vi "Stuckbead Scan and Auto Save_YCC.vi"(8 "File name add to the end":string="h0", 9 "Scan Range  (um)":dbl=2.0 format="%.3f", 10 "Save Data?":bool, 11 "Axis (XYZ)":enum16{"x", "y", "z"}(ring)) -> ()   [LabVIEW 2014]
uses:
  Main-Stage-PI/(Global) Current handle and LaserPower_YCC.vi
  <vilib>/Analysis/polynomials.llb/Scalar Polynomial Evaluation (DBL).vi
  <vilib>/Analysis/NI_AALPro.lvlib
panel:
  in  "Filter type":T1(ring)=enum."Moving-window avg"
  out "delta xBead (nm)":dbl[](array[numeric])
  out "Bead Position (nm)":dbl[](array[numeric])
  in  "Stuckbead path (dialog if empty)":path=path "D:/Calibration-Stuckbead-Scan/20181030/2/034619-x-Stuckbead Scan-20.00-step 5.00 nm-QPD height 0.814-h0.txt"
  in  "Who's Data":T2(ring)
  out "step size (nm)":dbl
  out "QPD height for tether (V)":dbl
  in  "Enum":enum16{"parity method", "max-min method"}(ring)=enum."max-min method"
  out "mean QPD":dbl
  out "Positon Start scan point (um)":dbl
  out "Filtered QPD data":dbl[](array[numeric])
  out "Filtered Stage Array":dbl[](array[numeric])
  out "Running time":dbl
  in  "Move to new Center?":bool=TRUE
  in  "no record \nscan rate  (um/s)":dbl=4.0
  out "need time":dbl
  out "True rate?":bool
  out "Sample points want to record":dbl
  out "Center (um)":dbl
  out "Move to":dbl
  in  "Tab Control":T3(tab)
  out "Filtered stage-QPD Graph (XY)":T4(graph)
  out "Raw+Filter stage-QPD Graph":cluster{"Raw Stage Array":dbl[], "data":dbl[]}[](graph)
  out "stage-QPD Graph":cluster{"Raw Stage Array":dbl[], "data":dbl[]}[](graph)
  in  "Avg points":i32=620
  out "Stage Array from one end to the other end":dbl[](array[numeric])
  out "total time to travel (s)":dbl
  out "Axis to Read":i32
  in  "T=+ first\nF=- first":bool
  out "Real initial position (um)":dbl format="%0.5f"
  in  "Sampling rate (Hz)":dbl=32000.0 format="%0.2f"
  in  "scan rate  (um/s)":dbl=1.0 format="%.3f"
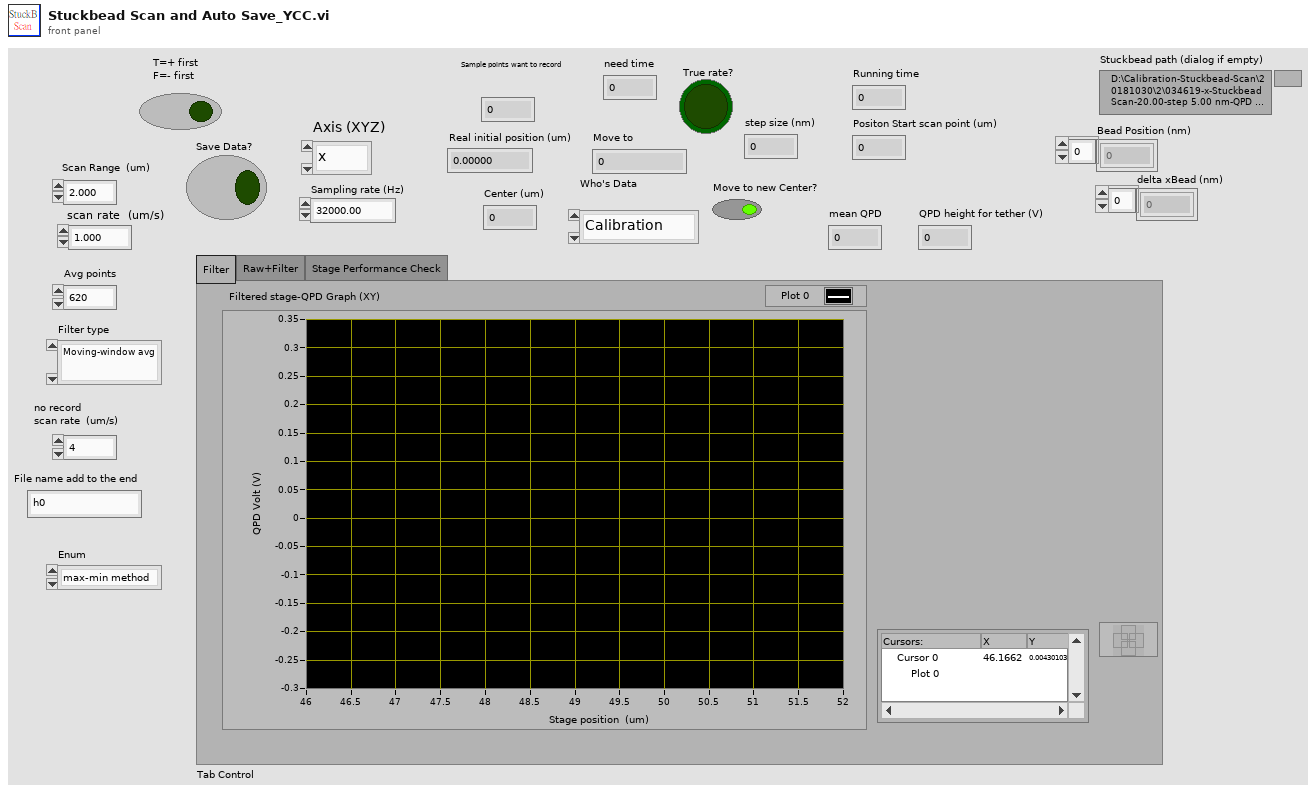
[diagram p1: front panel]
types:
  T1 = enum16{"Fixed-window avg", "Moving-window avg", "F+S-window avg", "S-G filter", "Fixed-window Median", "Moving-window Median "}
  T2 = enum16{"Calibration", "YCC", "PYW", "LCH", "YYH"}
  T3 = enum32{"Filter", "Raw+Filter", "Stage Performance Check"}
  T4 = cluster{"Filtered Stage Array":dbl[], "Another Axis Filt. QPD (X or Y)":dbl[]}[]
  T5 = cluster{"Raw Stage Array":dbl[], "Filtered QPD data out":dbl[]}
  T6 = cluster{"Filtered Stage Array":dbl[], "Filtered QPD data out":dbl[]}
  T7 = cluster{"Filtered Stage Array":dbl[], "Another Axis Filt. QPD (X or Y)":dbl[]}
  T8 = cluster{"Raw Stage Array":dbl[], "Filtered QPD data out":dbl[]}[]
  T9 = cluster{"stuckbead-QPD (V)":dbl[], "Bead radius (nm)":dbl[]}[]
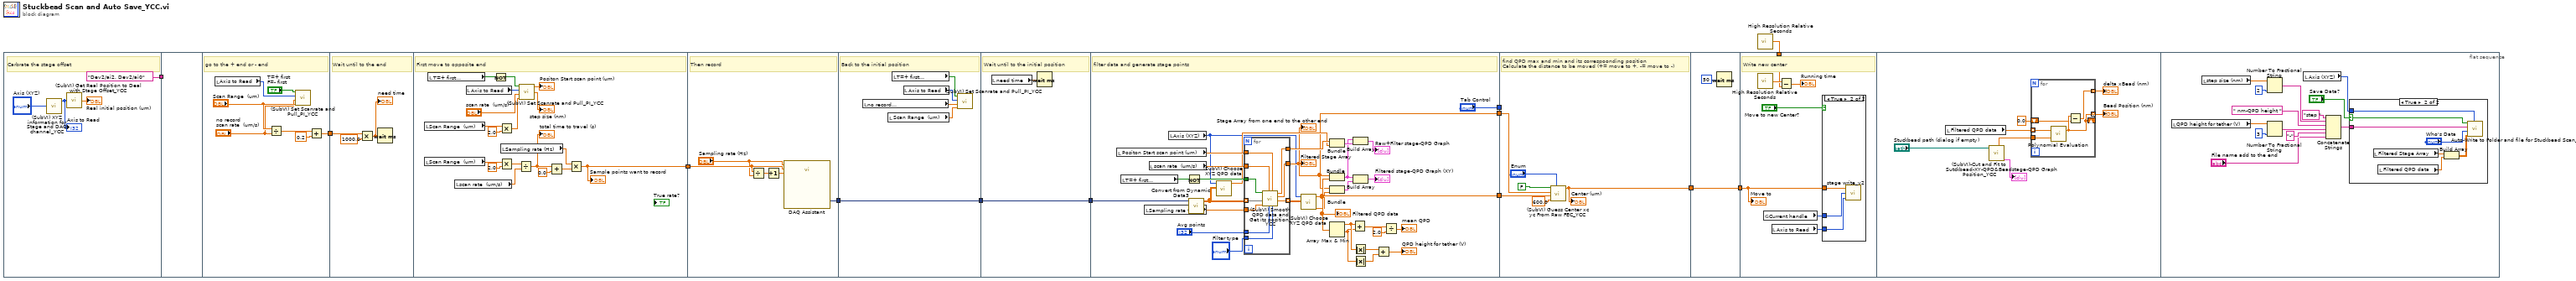
[diagram p0: block diagram]
diagram:
  n1 = flat-sequence {
    tunnel: [tag "Dev2/ai2, Dev2/ai0" ("physical channels")] -> w12
    tunnel: w12 -> [_]
    tunnel: [w19] -> w8
    tunnel: w8 -> [w26]
    tunnel: [w33] -> w5
    tunnel: [w49] -> w7
    tunnel: w5 -> [w48]
    tunnel: w7 -> [w54]
    tunnel: [w54] -> w6
    tunnel: w6 -> [w55]
    tunnel: [w55] -> w1
    tunnel: [w69] -> w11
    tunnel: [w66] -> w10
    tunnel: ["Tab Control"] -> w9
    tunnel: w1 -> [w59]
    tunnel: w11 -> [w99]
    tunnel: w10 -> [w102]
    tunnel: w9 -> [_]
    tunnel: [w98] -> w2
    tunnel: [w103] -> w3
    tunnel: w2 -> [w103]
    tunnel: w4 -> [w107]
    tunnel: w3 -> [w105]
    frame #0 {
      # "Carbrate the stage offset"
      n2 = call "(SubVI) XYZ information for Stage and DAQ channel_YCC.vi"("Axis  (Enum)"="Axis (XYZ)") -> ("Axis"=w13:i32)  [unwired: 3 in, 1 out]
      "Axis to Read" <- w13
      n3 = call "(SubVI) Get Real Position to Deal with Stage Offset_YCC.vi"("Axis"=w13) -> ("Real Current Commanded position (um)"=→"Real initial position (um)":dbl)  [unwired: 3 in, 1 out]
    }
    frame #1 {
    }
    frame #2 {
      # "go to the + end or - end"
      n4 = local read "Axis to Read"() -> (w23:i32)
      n5 = Divide(x="Scan Range  (um)", y="no record \nscan rate  (um/s)") -> (x/y=w21:dbl)
      n6 = call "(SubVI) Set Scanrate and Pull_PI_YCC.vi"("toward+ ?\nT=+, F=-"="T=+ first\nF=- first", "axis"=w23, "scan rate  (um/s)"="no record \nscan rate  (um/s)", "range  (um)"="Scan Range  (um)") -> ()  [unwired: 3 in, 2 out]
      n7 = Add(x=w21, y=0.2) -> (x+y=w19:dbl)
    }
    frame #3 {
      # "Wait until to the end"
      n8 = Multiply(x=w26, y=1000.0) -> (x*y=w24:dbl)
      "need time" <- w24
      n9 = Wait (ms)(milliseconds to wait=w24) -> ()  [unwired: 1 out]
    }
    frame #4 {
      # "First move to opposite end"
      n10 = local read "Scan Range  (um)"() -> (w30:dbl)
      n11 = local read "Scan Range  (um)"() -> (w35:dbl)
      n12 = local read "T=+ first\nF=- first"() -> (w31:bool)
      n13 = local read "scan rate  (um/s)"() -> (w34:dbl)
      n14 = local read "Axis to Read"() -> (w32:i32)
      n15 = Not(x=w31) -> (.not. x?=w41:bool)
      n16 = Multiply(x=w30, y=2.0) -> (x*y=w42:dbl)
      n17 = Multiply(x=w35, y=2.0) -> (x*y=w37:dbl)
      n18 = local read "Sampling rate (Hz)"() -> (w29:dbl)
      n19 = Divide(x=w37, y=w34) -> (x/y=w38:dbl)
      "total time to travel (s)" <- w38
      n20 = call "(SubVI) Set Scanrate and Pull_PI_YCC.vi"("toward+ ?\nT=+, F=-"=w41, "axis"=w32, "scan rate  (um/s)"="scan rate  (um/s)", "range  (um)"=w42) -> ("Start From  (um)"=→"Positon Start scan point (um)":dbl, "Traveling time (s)"=→"step size (nm)":dbl)  [unwired: 3 in]
      n21 = Add(x=w38, y=0.0) -> (x+y=w39:dbl)
      n22 = Multiply(x=w29, y=w39) -> (x*y=w33:dbl)
      "Sample points want to record" <- w33
    }
    frame #5 {
      # "Then record"
      n23 = Divide(x=w48, y="Sampling rate (Hz)") -> (x/y=w46:dbl)
      n24 = Increment(x=w46) -> (x+1=w45:dbl)
      n25 = call "DAQ Assistant"("rate"="Sampling rate (Hz)", "number of samples"=w48, "timeout (s)"=w45) -> ("data"=w49:dynamicdata)  [unwired: 14 in, 2 out]
    }
    frame #6 {
      # "Back to the initial position"
      n26 = local read "no record \nscan rate  (um/s)"() -> (w53:dbl)
      n27 = local read "Scan Range  (um)"() -> (w50:dbl)
      n28 = local read "T=+ first\nF=- first"() -> (w51:bool)
      n29 = local read "Axis to Read"() -> (w52:i32)
      n30 = call "(SubVI) Set Scanrate and Pull_PI_YCC.vi"("toward+ ?\nT=+, F=-"=w51, "axis"=w52, "scan rate  (um/s)"=w53, "range  (um)"=w50) -> ()  [unwired: 3 in, 2 out]
    }
    frame #7 {
      # "Wait until to the initial position"
      n31 = local read "need time"() -> (w56:dbl)
      n32 = Wait (ms)(milliseconds to wait=w56) -> ()  [unwired: 1 out]
    }
    frame #8 {
      # "filter data and generate stage points"
      n33 = local read "Positon Start scan point (um)"() -> (w78:dbl)
      n34 = local read "T=+ first\nF=- first"() -> (w80:bool)
      n35 = local read "Sampling rate (Hz)"() -> (w85:dbl)
      n36 = local read "scan rate  (um/s)"() -> (w84:dbl)
      n37 = local read "Axis (XYZ)"() -> (w64:enum16{"x", "y", "z"})
      n38 = Not(x=w80) -> (.not. x?=w79:bool)
      n39 = call "Convert from Dynamic Data3"("Dynamic Data Type"=w59) -> ("Array"=w58:dbl[][])  [unwired: 3 in]
      n40 = call "(SubVI) Choose XYZ QPD data.vi"("Filtered QPD data in"=w58, "Axis"=w64) -> ("Filtered QPD data out"=w68:dbl[])  [unwired: 8 in, 1 out]
      n41 = for {
        tunnel: w85 -> [w96]
        tunnel: w84 -> [w95]
        tunnel: "Avg points" -> [w94]
        tunnel: [w93] -> w66
        tunnel: [w92] -> w82
        tunnel: w79 -> [w91]
        tunnel: w78 -> [w90]
        tunnel: [w89] -> w65 mode=indexing
        tunnel: w58 -> [w88] mode=indexing
        tunnel: "Filter type" -> [w87]
        n42 = call "(SubVI) Smooth QPD data and Get its position_YCC.vi"("Filter type"=w87, "Initial position (um)"=w90, "Avg points"=w94, "scan rate  (um/s)"=w95, "Sampling rate (Hz)"=w96, "QPD data"=w88, "Direction\nT=+ \nF=-"=w91) -> ("Filtered QPD data"=w89:dbl[], "Filtered Stage Array"=w93:dbl[], "Raw Stage Array"=w92:dbl[])  [unwired: 2 in]
      }
      "Stage Array from one end to the other end" <- w66
      "Filtered Stage Array" <- w66
      n43 = call "(SubVI) Choose XYZ QPD data.vi"("Filtered QPD data in"=w65, "Axis"=w64) -> ("Another Axis Filt. QPD (X or Y)"=w63:dbl[], "Filtered QPD data out"=w69:dbl[])  [unwired: 8 in]
      "Filtered QPD data" <- w69
      n44 = Bundle("Raw Stage Array"=w82, "Filtered QPD data out"=w68) -> (w67:T5)  [unwired: 1 in]
      n45 = Bundle("Filtered Stage Array"=w66, "Filtered QPD data out"=w69) -> (w62:T6)  [unwired: 1 in]
      n46 = Bundle("Filtered Stage Array"=w66, "Another Axis Filt. QPD (X or Y)"=w63) -> (w61:T7)  [unwired: 1 in]
      n47 = Array Max & Min(array=w69) -> (max value=w74:dbl, min value=w73:dbl)  [unwired: 2 out]
      n48 = Add(x=w74, y=w73) -> (x+y=w77:dbl)
      n49 = Build Array(w62, w67) -> (→"Raw+Filter stage-QPD Graph":T8)
      n50 = Build Array(w62, w61) -> (→"Filtered stage-QPD Graph (XY)":T4)
      n51 = Absolute Value(x=w74) -> (abs(x)=w72:dbl)
      n52 = Absolute Value(x=w73) -> (abs(x)=w71:dbl)
      n53 = Add(x=w72, y=w71) -> (x+y=→"QPD height for tether (V)":dbl)
      n54 = Divide(x=w77, y=2.0) -> (x/y=→"mean QPD":dbl)
    }
    frame #9 {
      # "find QPD max and min and its correspoonding position\nCalculate the distance to be moved (+= move to +, -= move to -)"
      n55 = call "(SubVI) Guess Center xc yc From Raw FEC_YCC.vi"("Enum"="Enum", "avg range for QPD center (nm)"=600.0, "QPD array (V)"=w99, "Stage array(um)"=w102, "Read data?"=FALSE) -> ("Guess-stage-center(um)"=w98:dbl)  [unwired: 1 in, 3 out]
      "Center (um)" <- w98
    }
    frame #10 {
      n56 = Wait (ms)(milliseconds to wait=u32 50) -> ()  [unwired: 1 out]
    }
    frame #11 {
      # "Write new center"
      n57 = call <vilib>:"High Resolution Relative Seconds.vi"() -> ("relative seconds"=w108:dbl)
      n58 = global read "(Global) Current handle and LaserPower_YCC.vi" "Current handle"() -> (w110:i32)
      n59 = local read "Axis to Read"() -> (w109:i32)
      n60 = Subtract(x=w108, y=w107) -> (x-y=→"Running time":dbl)
      n61 = case shown="True" "Move to new Center?" {
        tunnel: w105 -> [_ w114]
        tunnel: w110 -> [_ w113]
        tunnel: w109 -> [_ w112]
        frame False {
        }
        frame True {
          n62 = call "stage write_v2.vi"("axis"=w112, "Incoming Handle"=w113, "position"=w114) -> ()  [unwired: 2 in, 1 out]
        }
      }
      "Move to" <- w105
    }
    frame #12 {
      n63 = local read "Filtered QPD data"() -> (w118:dbl[])
      n64 = call "(SubVI)-Cut and Fit to Sutckbead-XY-QPD&BeadPosition_YCC.vi"("Stuckbead path (dialog if empty)"="Stuckbead path (dialog if empty)") -> ("All fig"=→"stage-QPD Graph":T9, "Polynomial Coefficients\nx:QPD, y:BeadPos"=w119:dbl[])  [unwired: 2 in, 3 out]
      n65 = for {
        tunnel: w119 -> [w126]
        tunnel: w118 -> [w125] mode=indexing
        tunnel: [w124] -> w117 mode=indexing
        shift-right: [w124] -> _
        shift-left: 0.0 ("P(a)") -> [w123]
        tunnel: [w122] -> w116 mode=indexing
        n66 = call-poly <vilib>:"Polynomial Evaluation.vi"("P(x)"=w126, "a"=w125) -> ("P(a)"=w124:dbl)  [unwired: 1 out]
        n67 = Subtract(x=w124, y=w123) -> (x-y=w122:dbl)
      }
      "Bead Position (nm)" <- w117
      "delta xBead (nm)" <- w116
    }
    frame #13 {
      n68 = local read "QPD height for tether (V)"() -> (w132:dbl)
      n69 = local read "step size (nm)"() -> (w138:dbl)
      n70 = Number To Fractional String(number=w138, precision (6)=i16 2) -> (F-format string=w134:string)  [unwired: 2 in]
      n71 = Number To Fractional String(number=w132, precision (6)=i16 3) -> (F-format string=w130:string)  [unwired: 2 in]
      n72 = local read "Axis (XYZ)"() -> (w129:enum16{"x", "y", "z"})
      n73 = Concatenate Strings("step " ("string"), w134, " nm-QPD height " ("string"), w130, "-" ("string"), "File name add to the end") -> (w133:string)
      n74 = case shown="True" "Save Data?" {
        selector: "Save Data?" -> [_ w144]
        tunnel: w133 -> [_ w140]
        tunnel: w129 -> [_ w141]
        frame False {
        }
        frame True {
          n75 = local read "Filtered Stage Array"() -> (w146:dbl[])
          n76 = local read "Filtered QPD data"() -> (w145:dbl[])
          n77 = Build Array(w146, w145) -> (w143:dbl[][])
          n78 = call "Auto-Write to Folder and file for Stuckbead Scan_YCC.vi"("Axis (Enum)"=w141, "data to be saved"=w143, "Who's Data"="Who's Data", "File name add to the end"=w140, "Save?"=w144) -> ()  [unwired: 3 in, 2 out]
        }
      }
    }
  }
  n79 = call <vilib>:"High Resolution Relative Seconds.vi"() -> ("relative seconds"=w4:dbl)
